vi "fetch_and_translate_trigger.vi"(8 "error in (no error)":errorcluster, 11 "DisplayDL090216 in":refnum<class "DisplayDL090216.lvclass">) -> (0 "error out":errorcluster, 1 "sender TLC type":T2=enum."ImagingMode", 2 "internal trigger":T1, 3 "DisplayDL090216 out":refnum<class "DisplayDL090216.lvclass">)   [LabVIEW 2010, in "DisplayDL090216.lvclass"]
uses:
  DisplayDL090216.lvclass
  common/enumerations/top-level_component_type_enum.ctl
  action_enum.ctl
  GenericDisplay/GenericDisplay/trigger_enum.ctl
  common/classes/ErrorController/ErrorController/class_data.vi
  GenericDisplay/GenericDisplay/GenericDisplay.lvclass
  common/classes/ErrorController/ErrorController/ErrorController.lvclass
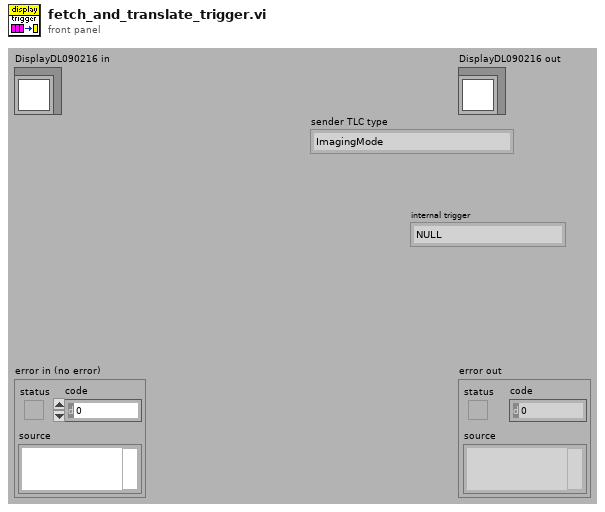
[diagram p1: front panel]
types:
  T1 = typedef "DisplayDL090216.lvclass/action_enum.ctl" = enum16{"NULL", "initialise", "terminate", "fetch", "process", "display", "register as observer"}
  T2 = typedef "top-level_component_type_enum.ctl" = enum16{"undefined", "ImagingMode", "ScanHead", "DAQ", "ImageAssembler", "Display", "DataCollection", "Analyser", "Stimulator", "ExperimentController", "Instrument", "Stage"}
  T3 = typedef "GenericDisplay.lvclass/trigger_enum.ctl" = enum8{"NULL", "display"}
  T4 = typedef "GenericToplevelComponent.lvclass/common_trigger_enum.ctl" = enum16{"NULL", "initialise", "terminate", "fetch command", "fetch data", "attach observer", "register as observer", "detach observer", "acknowledge", "start", "stop", "sweep started", "sweep finished", "experiment started", "experiment stopped"}
  T5 = typedef "trigger_type_enum.ctl" = enum8{"external", "internal", "common"}
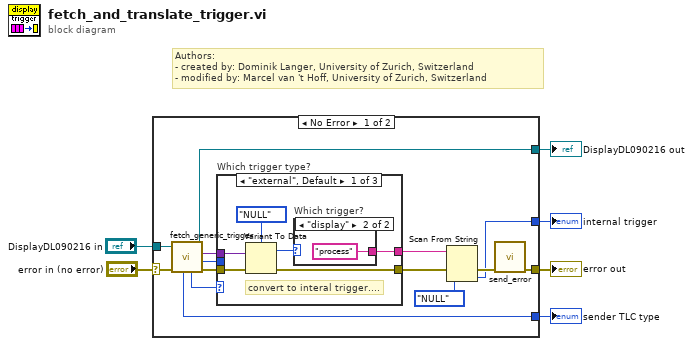
[diagram p0: block diagram]
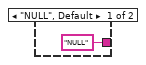
[diagram p2: hidden frame]
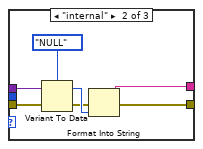
[diagram p3: hidden frame]
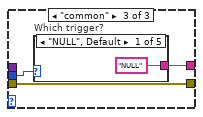
[diagram p4: hidden frame]
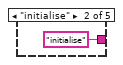
[diagram p5: hidden frame]
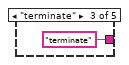
[diagram p6: hidden frame]
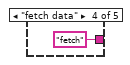
[diagram p7: hidden frame]
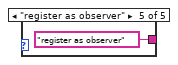
[diagram p8: hidden frame]
diagram:
  # "Authors: \n- created by: Dominik Langer, University of Zurich, Switzerland\n- modified by: Marcel van 't Hoff, University of Zurich, Switzerland"
  n1 = case shown="No Error" "error in (no error)" {
    selector: "error in (no error)" -> [w19 w45]
    tunnel: [w20 w45] -> w5
    tunnel: [w14 w44] -> w3
    tunnel: "DisplayDL090216 in" -> [w15 w44]
    tunnel: [w8 _] -> w1
    tunnel: [w12 _] -> w2
    frame No Error {
      n2 = call-dynamic "fetch_generic_trigger.vi"("error in (no error)"=w19, "GenericToplevelComponent in"=w15) -> ("error out"=w18:errorcluster, "common trigger"=w13:T4, "trigger"=w16:variant, "GenericToplevelComponent out"=w14:refnum<class "DisplayDL090216.lvclass">, "trigger type"=w17:T5, "sender TLC type"=w12:T2)  [unwired: 3 in, 1 out]
      n3 = case "Which trigger type?" shown="\"external\", Default" w17 {
        tunnel: [w26 w29 w38] -> w9
        tunnel: w18 -> [w23 w34 w38]
        tunnel: w16 -> [w22 w35 _]
        tunnel: w13 -> [_ _ w37]
        tunnel: [w21 w31 w36] -> w7
        frame "external", Default {
          # "convert to interal trigger...."
          n4 = Variant To Data(error in=w23, Variant=w22, type=trigger_enum."NULL" ("trigger")) -> (error out=w26:errorcluster, data=w25:T3)
          n5 = case "Which trigger?" shown="\"display\"" w25 {
            tunnel: ["NULL" "process"] -> w21
            frame "NULL", Default {
            }
            frame "display" {
            }
          }
        }
        frame "internal" {
          n6 = Variant To Data(error in=w34, Variant=w35, type=action_enum."NULL" ("internal trigger")) -> (error out=w30:errorcluster, data=w32:T1)
          n7 = Format Into String(error in=w30, w32) -> (resulting string=w31:string, error out=w29:errorcluster)  [unwired: 2 in]
        }
        frame "common" {
          n8 = case "Which trigger?" shown="\"NULL\", Default" w37 {
            tunnel: ["NULL" "initialise" "terminate" "fetch" "register as observer"] -> w36
            frame "NULL", Default {
            }
            frame "initialise" {
            }
            frame "terminate" {
            }
            frame "fetch data" {
            }
            frame "register as observer" {
            }
          }
        }
      }
      n9 = Scan From String(input string=w7, error in=w9, default 1=action_enum."NULL" ("internal trigger")) -> (error out=w10:errorcluster, output 1=w8:T1)  [unwired: 2 in, 2 out]
      n10 = call "send_error.vi"("error in (no error)"=w10) -> ("error out"=w20:errorcluster)  [unwired: 10 in]
    }
    frame Error {
    }
  }
  "error out" <- w5
  "DisplayDL090216 out" <- w3
  "sender TLC type" <- w2
  "internal trigger" <- w1
